vi "VAT_valve_adjust_setpoint.vi"(0 "VAT Valve COM port":refnum<visa-resource-name>, 1 "Flow":dbl, 3 "Pressure":dbl, 5 "Operating Mode":u16(ring) items=["Pressure", "Flow"], 9 "Unit":string, 11 "error in (no error)":errorcluster) -> (4 "VAT Valve COM port out":refnum<visa-resource-name>, 15 "error out":errorcluster)   [LabVIEW 2019]
uses:
  <vilib>/regexp/Match Regular Expression.xnode
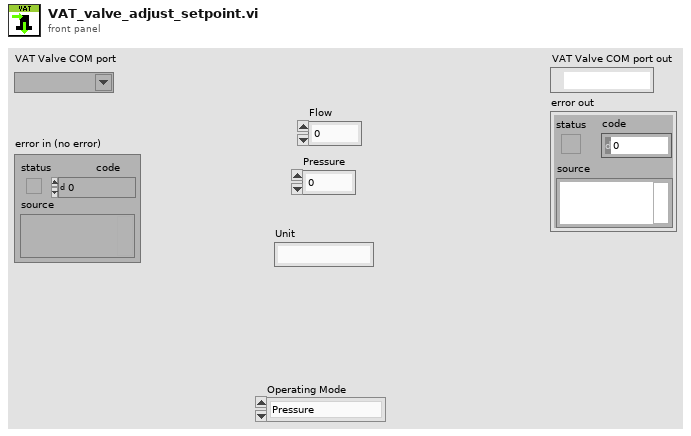
[diagram p1: front panel]
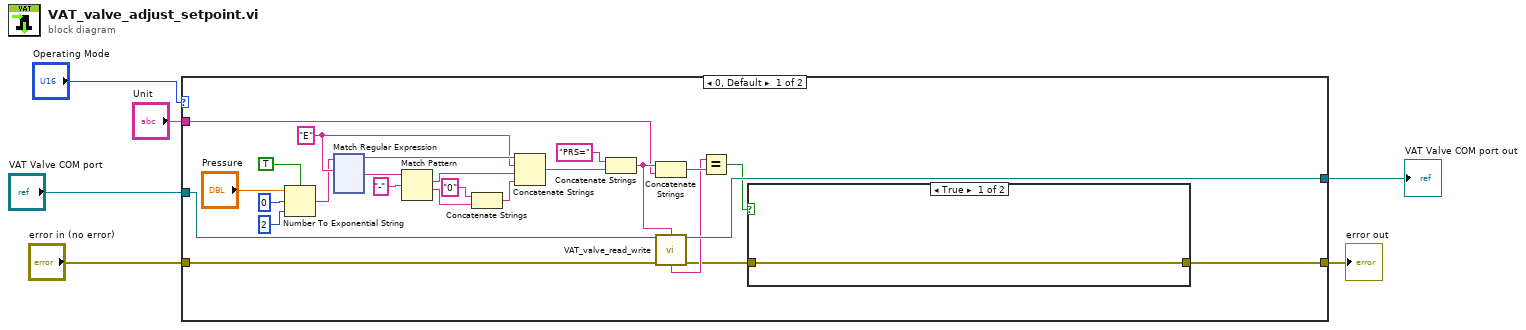
[diagram p0: block diagram]
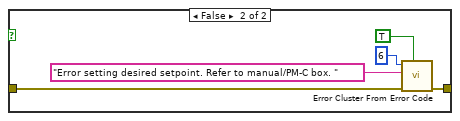
[diagram p2: hidden frame]
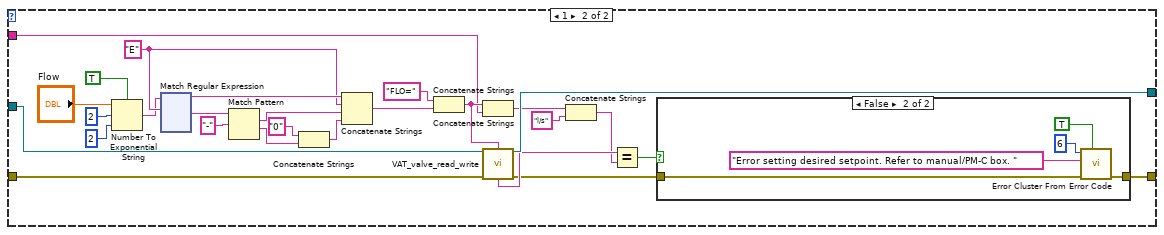
[diagram p3: hidden frame]
diagram:
  n1 = case shown="0, Default" "Operating Mode" {
    tunnel: "VAT Valve COM port" -> [w31 w178]
    tunnel: "error in (no error)" -> [w30 w177]
    tunnel: [w24 w171] -> w3
    tunnel: "Unit" -> [w22 w169]
    tunnel: [w17 w162] -> w1
    frame 0, Default {
      w11 = "E" ("regular expression")
      n2 = Number To Exponential String(number="Pressure", precision (6)=i16 2, 1:TRUE ("use system decimal point (T)"), 3:i16 0 ("width (-)")) -> (E-format string=w8:string)
      n3 = xnode "Match Regular Expression"("input string"=w8, "regular expression"=w11) -> ("before match"=w12:string, "after match"=w16:string)  [unwired: 4 in, 3 out]
      n4 = Match Pattern(string=w16, regular expression="-") -> (match substring=w10:string, after substring=w14:string)  [unwired: 1 in, 2 out]
      n5 = Concatenate Strings("0", w14) -> (w9:string)
      n6 = Concatenate Strings(w12, w11, w10, w9) -> (w7:string)
      n7 = Concatenate Strings("PRS=" ("string"), w7) -> (w23:string)
      n8 = Concatenate Strings(w23, w22) -> (w21:string)
      n9 = call "VAT_valve_read_write.vi"("VAT Valve COM port"=w31, "Write String"=w23, "error in (no error)"=w30) -> ("VAT Valve COM port out"=w24:refnum<visa-resource-name>, "Read String"=w20:string, "error out"=w18:errorcluster)  [unwired: 10 in]
      n10 = Equal?(x=w20, y=w21) -> (x = y?=w19:bool)
      n11 = case shown="True" w19 {
        tunnel: w18 -> [w146 w151]
        tunnel: [w146 w147] -> w17
        frame True {
        }
        frame False {
          n12 = call <vilib>:"Error Cluster From Error Code.vi"("show call chain? (False)"=TRUE, "error in (no error)"=w151, "error message (\"\")"="Error setting desired setpoint. Refer to manual/PM-C box. " ("error message (\"\")"), "error code (0)"=6) -> ("error out"=w147:errorcluster)  [unwired: 5 in]
        }
      }
    }
    frame 1 {
      w156 = "E" ("regular expression")
      n13 = Number To Exponential String(number="Flow", precision (6)=i16 2, 1:TRUE ("use system decimal point (T)"), 3:i16 2 ("width (-)")) -> (E-format string=w153:string)
      n14 = xnode "Match Regular Expression"("input string"=w153, "regular expression"=w156) -> ("before match"=w157:string, "after match"=w161:string)  [unwired: 4 in, 3 out]
      n15 = Match Pattern(string=w161, regular expression="-") -> (match substring=w155:string, after substring=w159:string)  [unwired: 1 in, 2 out]
      n16 = Concatenate Strings("0", w159) -> (w154:string)
      n17 = Concatenate Strings(w157, w156, w155, w154) -> (w152:string)
      n18 = Concatenate Strings("FLO=" ("string"), w152) -> (w170:string)
      n19 = Concatenate Strings(w170, w169) -> (w165:string)
      n20 = call "VAT_valve_read_write.vi"("VAT Valve COM port"=w178, "Write String"=w170, "error in (no error)"=w177) -> ("VAT Valve COM port out"=w171:refnum<visa-resource-name>, "Read String"=w168:string, "error out"=w166:errorcluster)  [unwired: 10 in]
      n21 = Concatenate Strings(w165, "l/s" ("string")) -> (w163:string)
      n22 = Equal?(x=w168, y=w163) -> (x = y?=w167:bool)
      n23 = case shown="False" w167 {
        tunnel: w166 -> [w293 w298]
        tunnel: [w293 w294] -> w162
        frame True {
        }
        frame False {
          n24 = call <vilib>:"Error Cluster From Error Code.vi"("show call chain? (False)"=TRUE, "error in (no error)"=w298, "error message (\"\")"="Error setting desired setpoint. Refer to manual/PM-C box. " ("error message (\"\")"), "error code (0)"=6) -> ("error out"=w294:errorcluster)  [unwired: 5 in]
        }
      }
    }
  }
  "VAT Valve COM port out" <- w3
  "error out" <- w1
